vi "CPP_SpectraFit.vi"() -> (5 "Plug in titles":string[](array[string]), 7 "Plug in values":string[](array[string]))   [LabVIEW 2020]
uses:
  <vilib>/Analysis/2dsp.llb/Integral Method.ctl
  Controls/Instrument_Array.ctl
  Controls/Post_Process.ctl
  Controls/Graph_Type.ctl
  <vilib>/Analysis/8numeric.llb/1D Numeric Integration.vi
  Globals/Meas_global.vi
  <vilib>/Analysis/NI_AALPro.lvlib
  <vilib>/Analysis/NI_AALBase.lvlib
panel:
  out "Av Sampling Rate":dbl
  out "mean":dbl format="%0.2f"
  out "variance":dbl format="%.4f"
  out "Integral":dbl format="%0.4f"
  in  "integration method":T1 items=["Trapezoidal Rule", "Simpson's Rule", "Simpson's 3/8 Rule", "Bode Rule"]
  in  "Divider":i32(slide)=10 scale=1.0..100000.0 scale format="%#_6e"
  out "dF/ Hz":dbl
  in  "Show Smooth":bool=TRUE
  in  "Save Spectra?":bool
  in  "Desired number of samples per block":i32=32768
  out "Spectra":cluster{"Frequencies":dbl[], dbl[]}[](graph)
  in  "Averaging samples":i32=1 min=1 max=1000
  in  "Spectra Index (from ALL channels)":i32
  out "Waveform Graph":dbl[][](graph)
  in  "Channels to Plot":i32[](array[ring])=[0] items=["Pitot (URef)", "Mano (5HP1)", "Mano (5HP2)", "Mano (5HP3)", "Mano (5HP4)", "Mano (5HP5)", "HW (Uhf)", "Save Nothing"]
  # "Run this VI to update the channel names"
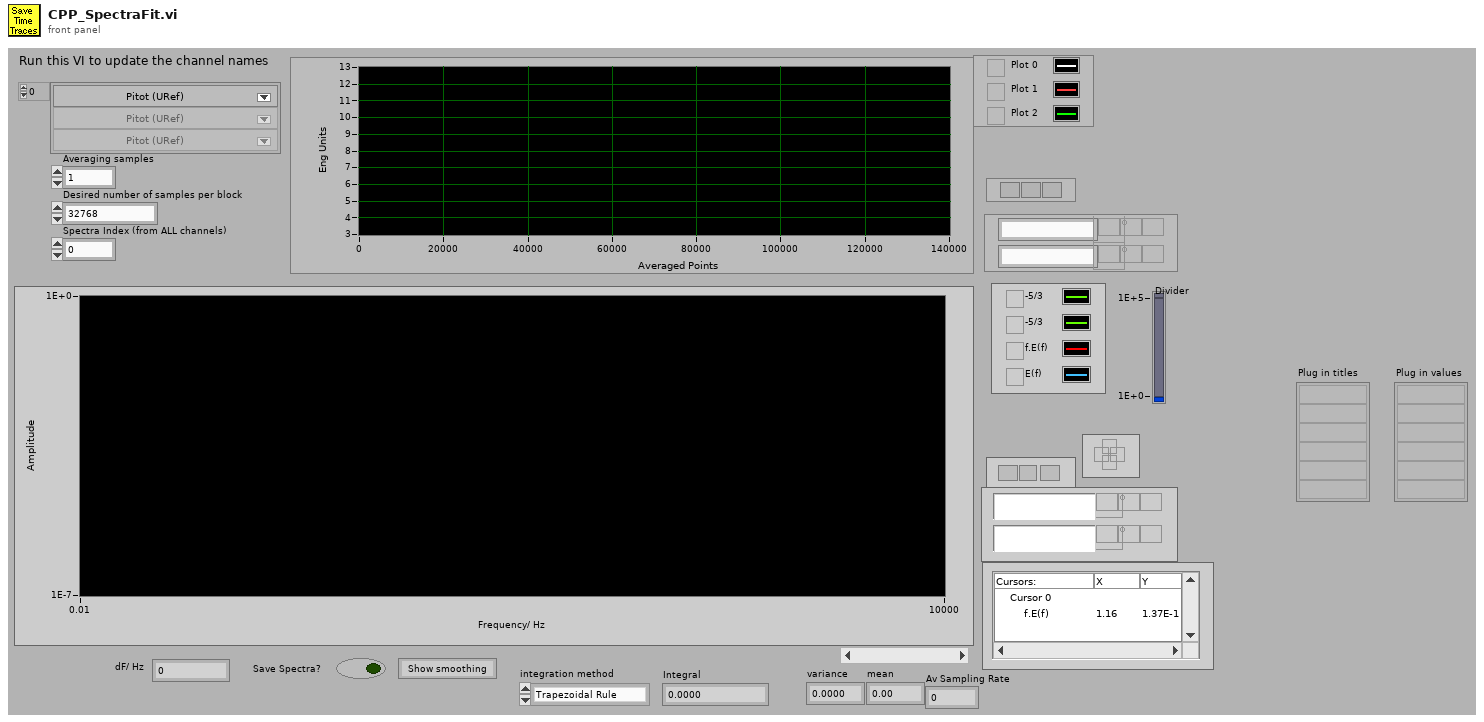
[diagram p1: front panel]
types:
  T1 = typedef "NI_AALPro.lvlib/Integral Method.ctl" = i32
  T2 = typedef "Analysis_info_cluster.ctl" = cluster{"Colour":u32, "Inst type":T3, "Inst name":string, "Symbol":string, "Code name":string, "Extra Info":string, "Inst Array":T4, "Extra Titles":string[], "Extra Values":string[], "U":dbl, "u^2":dbl, "u^3":dbl, "u^4":dbl, "Skew_u":dbl, "Kurt_u":dbl, "Sd Error in Mean":dbl, "% u'/U":dbl, "X":dbl, "Y":dbl, "Z":dbl, "Timescale integral Estimate":dbl, "Sd Error in Variance":dbl, "Calib File":path, "Calib Constants":dbl[], "Output Position":bool, "Stats":enum16{"None", "Basic", "Full"}, "Av Sampling Rate":dbl, "Av No of Samples":dbl, "Total Meas Time (s)":dbl, "ADAM Ch Name":string, "Max value":dbl, "Min value":dbl, "Req Sample Rate Hz":dbl, "Sync Delay Time (s)":dbl, "Ch No":i16, "Device":string, "Use Latest Calib":bool, "Port":string, "Metadata Ch Names":string[], "Metadata Ch Values":string[]}
  T3 = typedef "Inst_type.ctl" = enum16{"Propeller anemometer", "Raw voltage", "Pressure Transducer", "Pitot-static tube", "Preston tube", "Hot wire", "Cross wire 1", "Cross wire 2", "Generic Linear", "Generic Polynomial", "Generic BackPoly", "Fast FID", "Thermocouple", "Cold wire", "Pulsed Wire", "LDA Vel", "LDA Tran time", "LDA Arr time", "Microphone"}
  T4 = typedef "Instrument_Array.ctl" = enum16{"PWA", "LDA", "Analogue"}
  T5 = typedef "Post_Process.ctl" = enum16{"Take New Data", "Post Process Raw Data File"}
  T6 = typedef "Graph_Type.ctl" = enum16{"Show no graph", "Voltage trace", "Velocity trace", "Vel histogram", "Spectrum", "f.E(f) v Log f", "Auto-Corr"}
  T7 = cluster{"Plot 1":u16, "Plot 2":u16, "Save graph":u16, "Plot Type":T6}
  T8 = typedef "Time_Trace_Cluster.ctl" = cluster{"Weighting":dbl[], "Time (s)":dbl[], "Voltage":dbl[], "Eng Values":dbl[]}
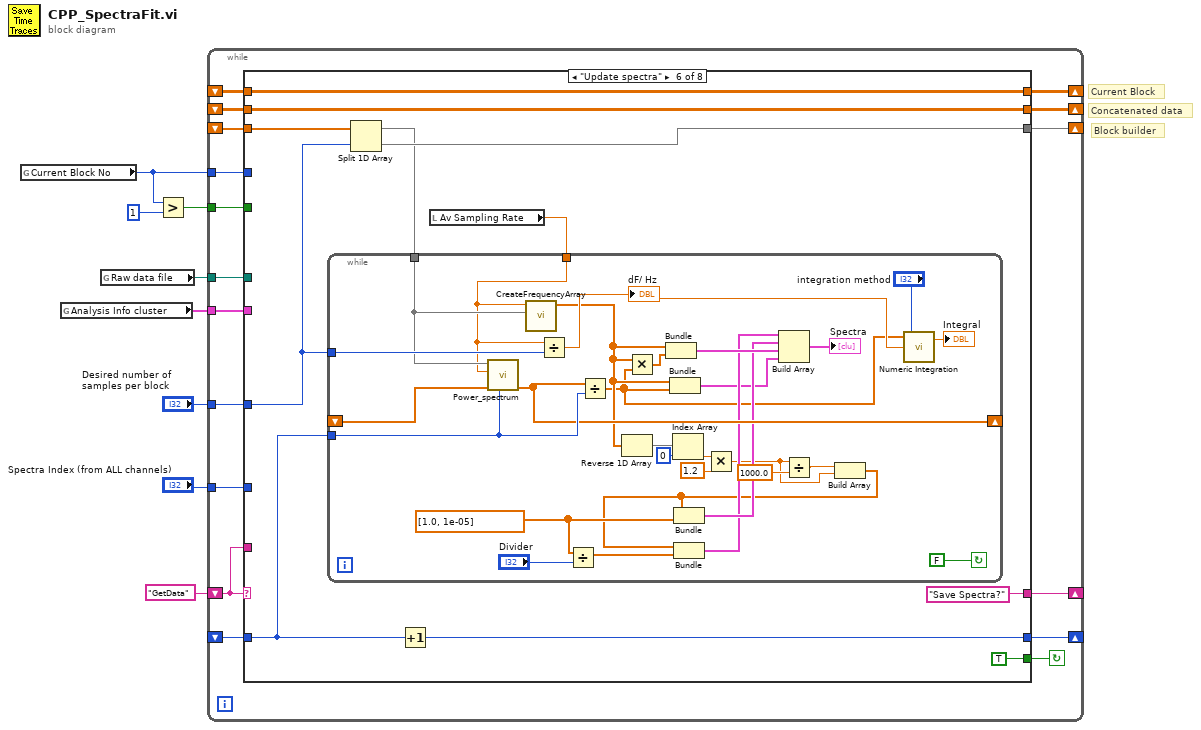
[diagram p0: block diagram]
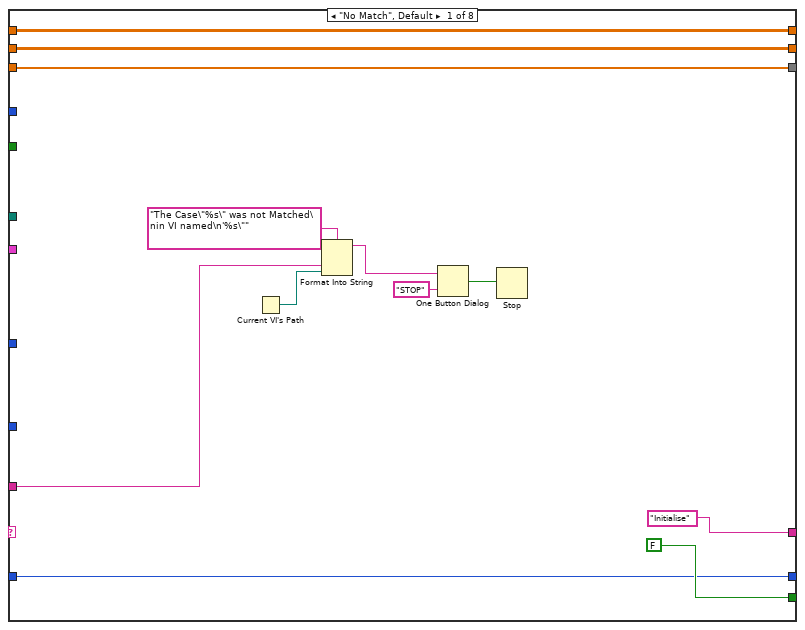
[diagram p2: hidden frame]
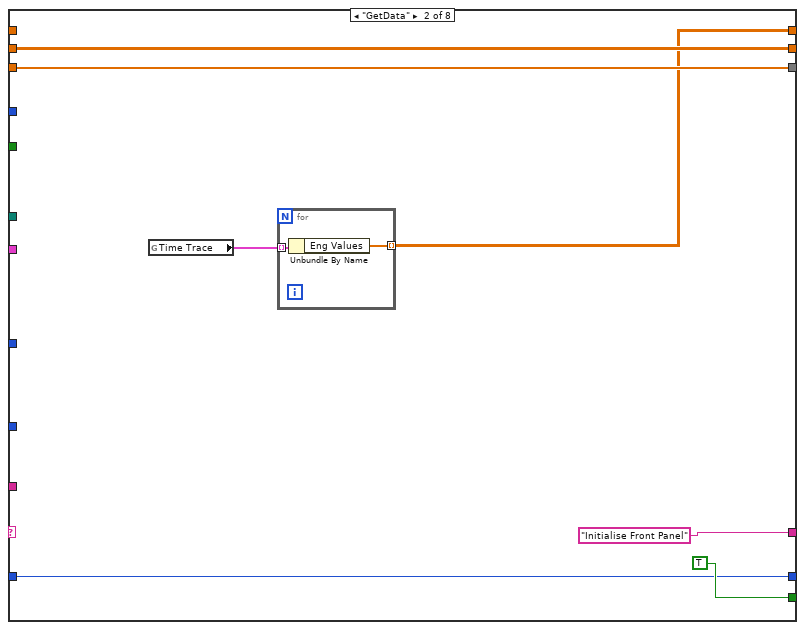
[diagram p3: hidden frame]
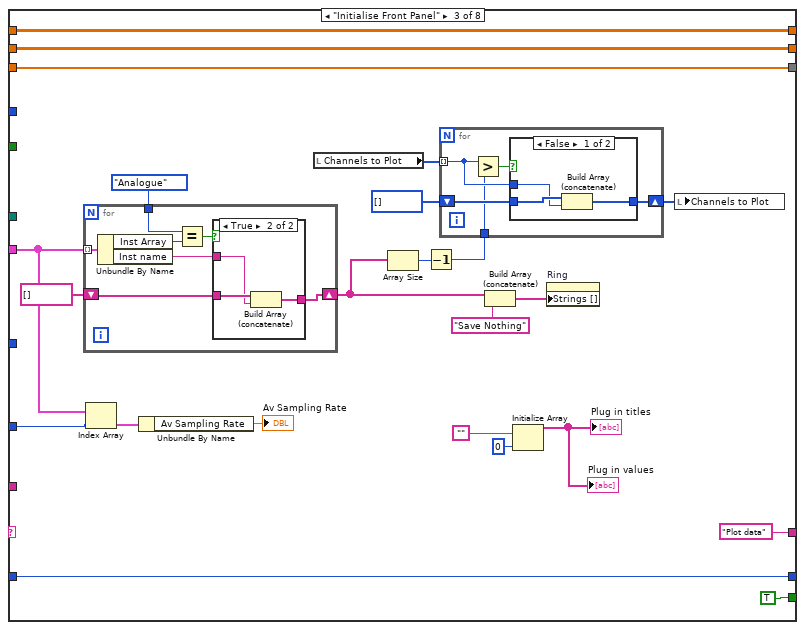
[diagram p4: hidden frame]
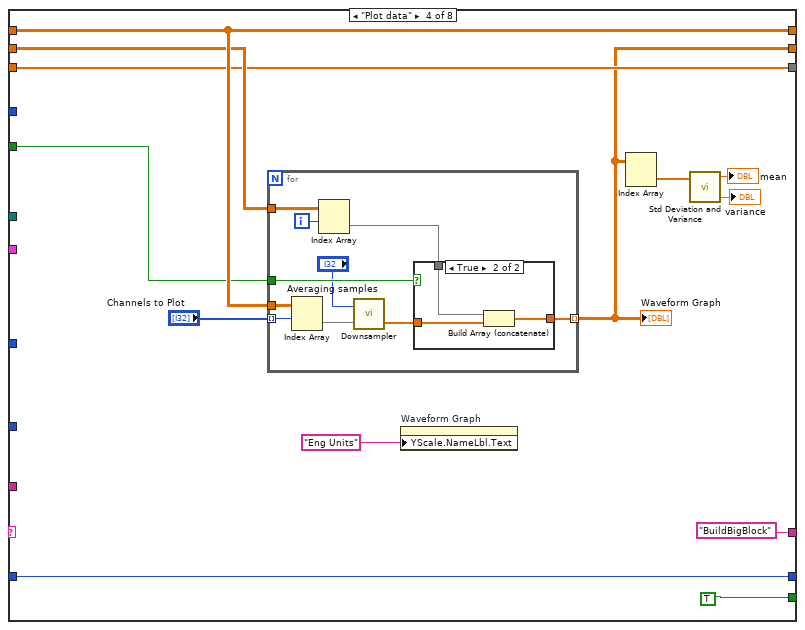
[diagram p7: hidden frame]
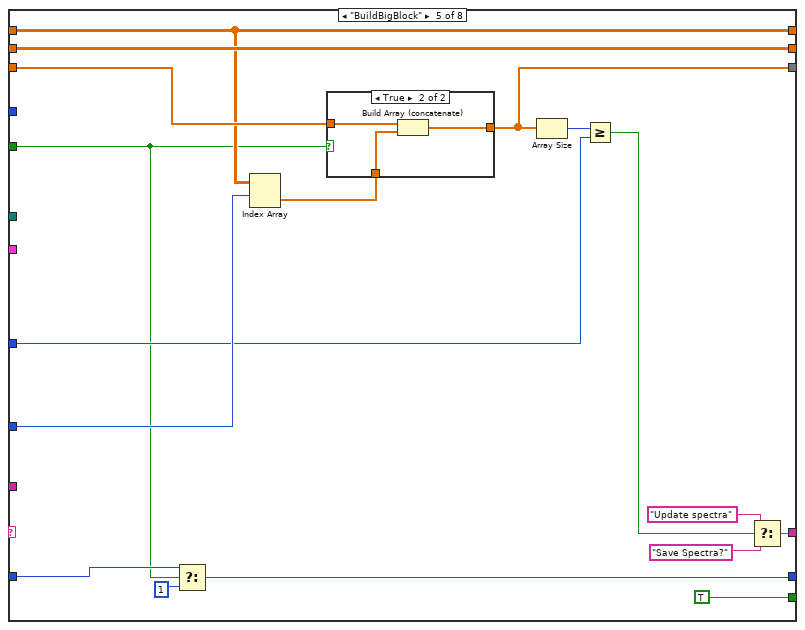
[diagram p9: hidden frame]
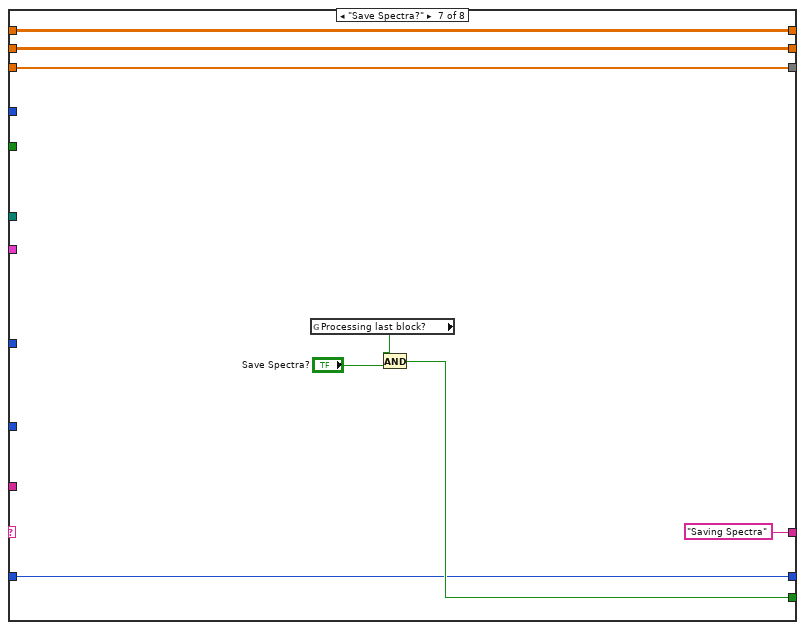
[diagram p11: hidden frame]
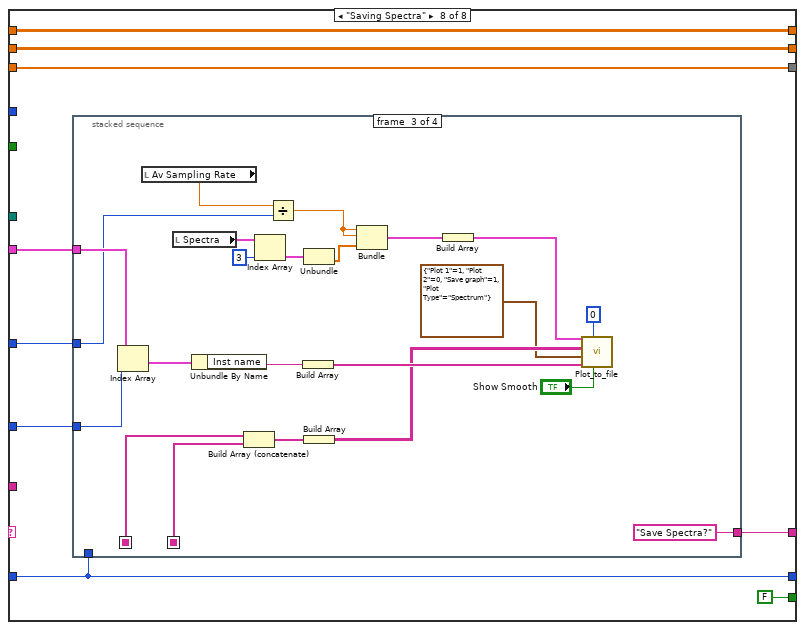
[diagram p12: hidden frame]
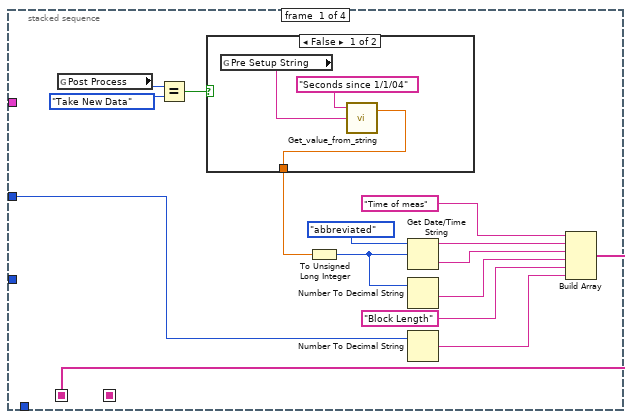
[diagram p13: hidden frame]
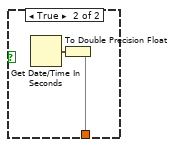
[diagram p14: hidden frame]
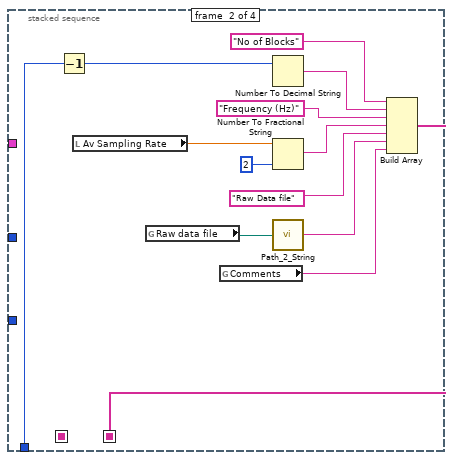
[diagram p15: hidden frame]
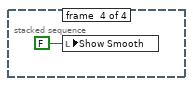
[diagram p16: hidden frame]
diagram:
  # "Block builder"
  # "Concatenated data"
  # "Current Block"
  n1 = global read "Meas_global.vi" "Current Block No"() -> (w5:i32)
  n2 = global read "Meas_global.vi" "Analysis Info cluster"() -> (w4:T2[])
  n3 = global read "Meas_global.vi" "Raw data file"() -> (w7:path)
  n4 = Greater?(x=w5, y=1) -> (0:w3:bool)
  n5 = while {
    shift-left: "GetData" -> [w23]
    shift-right: [w24] -> _
    tunnel: w7 -> [w22]
    tunnel: w3 -> [w21]
    tunnel: w5 -> [w20]
    tunnel: w4 -> [w19]
    shift-right: [w18] -> _
    shift-left: _ -> [w17]
    shift-right: [w15] -> _
    shift-left: _ -> [w16]
    shift-right: [w13] -> _
    shift-left: _ -> [w14]
    tunnel: "Desired number of samples per block" -> [w12]
    tunnel: "Spectra Index (from ALL channels)" -> [w11]
    shift-right: [w10] -> _
    shift-left: _ -> [w9]
    stop <- w25 continue-if-true
    n6 = case shown="\"Update spectra\"" w23 {
      tunnel: [FALSE TRUE TRUE TRUE ("Calculate Spectra and Histogram?") TRUE ("Calculate Spectra and Histogram?") TRUE ("Calculate Spectra and Histogram?") w179 FALSE ("Calculate Spectra and Histogram?")] -> w25
      tunnel: ["Initialise" "Initialise Front Panel" "Plot data" "BuildBigBlock" ("t") w118 "Save Spectra?" "Saving Spectra" w192] -> w24
      tunnel: w23 -> [w32 _ _ _ _ _ _ _]
      tunnel: w22 -> [_ _ _ _ _ _ _ _]
      tunnel: w21 -> [_ _ _ w100 w121 _ _ _]
      tunnel: w20 -> [_ _ _ _ _ _ _ _]
      tunnel: w19 -> [_ _ w50 _ _ _ _ w190]
      tunnel: [w29 w38 w59 w102 w131 w147 w184 w193] -> w18
      tunnel: w17 -> [w29 _ w59 w102 w131 w147 w184 w193]
      tunnel: w16 -> [w28 w42 w58 w101 w132 w148 w185 w194]
      tunnel: [w28 w42 w58 w93 w132 w148 w185 w194] -> w15
      tunnel: w14 -> [w27 w41 w55 w97 w133 w146 w182 w191]
      tunnel: [w27 w41 w55 w97 w129 w145 w182 w191] -> w13
      tunnel: w12 -> [_ _ _ _ w125 w141 _ w187]
      tunnel: w11 -> [_ _ w49 _ w127 _ _ w189]
      tunnel: [w26 w40 w54 w96 w122 w139 w178 w186] -> w10
      tunnel: w9 -> [w26 w40 w54 w96 w123 w140 w178 w186]
      frame "No Match", Default {
        n7 = Current VI's Path() -> (path=w31:path)
        n8 = Format Into String(format string="The Case\"%s\" was not Matched\nin VI named\n'%s\"" ("Format String"), w32, w31) -> (resulting string=w35:string)  [unwired: 2 in, 1 out]
        n9 = One Button Dialog(message=w35, button name ("OK")="STOP") -> (true=w33:bool)
        n10 = Stop(stop? (T)=w33) -> ()
      }
      frame "GetData" {
        n11 = global read "Meas_global.vi" "Time Trace"() -> (w39:T8[])
        n12 = for {
          tunnel: w39 -> [w46] mode=indexing
          tunnel: [w45] -> w38 mode=indexing
          n13 = Unbundle By Name(w46) -> ("Eng Values"=w45:dbl[])
        }
      }
      frame "Initialise Front Panel" {
        n14 = for {
          tunnel: Instrument_Array."Analogue" ("Inst Array") -> [w75]
          tunnel: w50 -> [w74] mode=indexing
          shift-right: [w71] -> w53
          shift-left: string[] [] -> [w72]
          n15 = Unbundle By Name(w74) -> ("Inst Array"=w76:T4, "Inst name"=w70:string)
          n16 = Equal?(x=w75, y=w76) -> (x = y?=w73:bool)
          n17 = case shown="True" w73 {
            tunnel: w72 -> [w77 w80]
            tunnel: [w77 w79] -> w71
            tunnel: w70 -> [_ w78]
            frame False {
            }
            frame True {
              n18 = Build Array (concatenate)(w80, w78) -> (w79:string[])
            }
          }
        }
        n19 = Index Array(array=w50, index=w49) -> (element=w48:T2)
        n20 = Unbundle By Name(w48) -> ("Av Sampling Rate"=→"Av Sampling Rate":dbl)
        n21 = local read "Channels to Plot"() -> (w66:i32[])
        n22 = Array Size(array=w53) -> (size(s)=w61:i32)
        n23 = Decrement(x=w61) -> (x-1=w60:i32)
        n24 = for {
          tunnel: w66 -> [w82] mode=indexing
          shift-right: [w83] -> w64
          shift-left: i32[] [] -> [w84]
          tunnel: w60 -> [w81]
          n25 = Greater?(x=w82, y=w81) -> (0:w85:bool)
          n26 = case shown="False" w85 {
            tunnel: w84 -> [w88 w89]
            tunnel: [w87 w89] -> w83
            tunnel: w82 -> [w86 _]
            frame False {
              n27 = Build Array (concatenate)(w88, w86) -> (w87:i32[])
            }
            frame True {
            }
          }
        }
        n28 = Build Array (concatenate)(w53, "Save Nothing") -> (w62:string[])
        n29 = Initialize Array("", 0) -> (→"Plug in values" →"Plug in titles":string[])
        n30 = property on="Ring" class="Ring (strict)"("Strings []"=w62) -> ()  [unwired: 2 in, 2 out]
        n31 = local write "Channels to Plot"(w64) -> ()
      }
      frame "Plot data" {
        n32 = for {
          tunnel: w102 -> [w112]
          tunnel: "Channels to Plot" -> [w111] mode=indexing
          tunnel: w101 -> [w108]
          tunnel: [w109] -> w93 mode=indexing
          tunnel: w100 -> [w110]
          i -> [w107]
          n33 = Index Array(array=w112, index (row)=w111) -> (element=w105:dbl[])  [unwired: 1 in]
          n34 = Index Array(array=w108, index (row)=w107) -> (element=w106:dbl[])  [unwired: 1 in]
          n35 = call "Downsampler.vi"("Input Array"=w105, "Averaging samples"="Averaging samples") -> ("Downsampled Array"=w104:dbl[])  [unwired: 1 out]
          n36 = case shown="True" w110 {
            tunnel: w106 -> [_ w116]
            tunnel: w104 -> [w113 w115]
            tunnel: [w113 w114] -> w109
            frame False {
            }
            frame True {
              n37 = Build Array (concatenate)(w116, w115) -> (w114:dbl[])
            }
          }
        }
        "Waveform Graph" <- w93
        n38 = property on="Waveform Graph" class="WFGraph (strict)"("YScale.NameLbl.Text"="Eng Units") -> ()  [unwired: 2 in, 2 out]
        n39 = Index Array(array=w93) -> (element=w92:dbl[])  [unwired: 2 in]
        n40 = call <vilib>:"Std Deviation and Variance.vi"("X"=w92) -> ("mean"=→"mean":dbl, "variance"=→"variance":dbl)  [unwired: 1 in, 1 out]
      }
      frame "BuildBigBlock" {
        n41 = Select(t=w123, s=w121, f=1) -> (s? t:f=w122:i32)
        n42 = Index Array(array=w131, index (row)=w127) -> (element=w130:dbl[])  [unwired: 1 in]
        n43 = case shown="True" w121 {
          tunnel: w133 -> [_ w137]
          tunnel: [w134 w136] -> w129
          tunnel: w130 -> [w134 w135]
          frame False {
          }
          frame True {
            n44 = Build Array (concatenate)(w137, w135) -> (w136:dbl[])
          }
        }
        n45 = Array Size(array=w129) -> (size(s)=w128:i32)
        n46 = Greater Or Equal?(x=w128, y=w125) -> (x >= y?=w117:bool)
        n47 = Select(t="Update spectra", s=w117, f="Save Spectra?") -> (s? t:f=w118:string)
      }
      frame "Update spectra" {
        n48 = Split 1D Array(array=w146, index=w141) -> (first subarray=w142:dbl[], second subarray=w145:dbl[])
        n49 = Increment(x=w140) -> (x+1=w139:i32)
        n50 = local read "Av Sampling Rate"() -> (w138:dbl)
        n51 = while {
          shift-left: _ -> [w173]
          shift-right: [w174] -> _
          tunnel: w142 -> [w172]
          tunnel: w140 -> [w176]
          tunnel: w141 -> [w175]
          tunnel: w138 -> [w149]
          stop <- FALSE continue-if-true
          w167 = dbl[] [1.0, 1e-05]
          n52 = call "Power_spectrum.vi"("Block No"=w176, "Spectrum input array"=w173, "Sampling frequency"=w149, "U"=w172) -> ("Spectrum Accumulator array"=w174:dbl[])  [unwired: 1 in, 3 out]
          n53 = call "CreateFrequencyArray.vi"("Signal"=w172, "Actual Sampling rate (Hz)"=w149) -> ("Frequencies"=w153:dbl[])  [unwired: 9 in]
          n54 = Divide(x=w149, y=w175) -> (x/y=w154:dbl)
          "dF/ Hz" <- w154
          n55 = Divide(x=w167, y="Divider") -> (x/y=w168:dbl[])
          n56 = Divide(x=w174, y=w176) -> (x/y=w150:dbl[])
          n57 = Reverse 1D Array(array=w153) -> (reversed array=w162:dbl[])
          n58 = Multiply(x=w153, y=w150) -> (x*y=w164:dbl[])
          n59 = Bundle("Frequencies"=w153, w164) -> (w170:cluster{"Frequencies":dbl[], dbl[]})  [unwired: 1 in]
          n60 = Bundle("Frequencies"=w153, w150) -> (w163:cluster{"Frequencies":dbl[], dbl[]})  [unwired: 1 in]
          n61 = Index Array(array=w162, index=0) -> (element=w160:dbl)
          n62 = Multiply(x=w160, y=1.2) -> (x*y=w156:dbl)
          n63 = Divide(x=w156, y=1000.0) -> (x/y=w157:dbl)
          n64 = Build Array(w157, w156) -> (w155:dbl[])
          n65 = Bundle(w155, w167) -> (w169:cluster{dbl[], dbl[]})  [unwired: 1 in]
          n66 = Bundle(w155, w168) -> (w165:cluster{dbl[], dbl[]})  [unwired: 1 in]
          n67 = Build Array(w165, w169, w170, w163) -> (→"Spectra":cluster{"Frequencies":dbl[], dbl[]}[])
          n68 = call-poly <vilib>:"Numeric Integration.vi"("integration method"="integration method", "dt"=w154, "Input Array"=w150) -> ("result"=→"Integral":dbl)  [unwired: 1 out]
        }
      }
      frame "Save Spectra?" {
        n69 = global read "Meas_global.vi" "Processing last block?"() -> (w180:bool)
        n70 = And(x=w180, y="Save Spectra?") -> (x .and. y?=w179:bool)
      }
      frame "Saving Spectra" {
        n71 = stacked-sequence {
          seq-local: [w198 _ _ _] -> [_ _ w240 _]
          seq-local: [_ w219 _ _] -> [_ _ w239 _]
          tunnel: [_ _ "Save Spectra?" _] -> w192
          tunnel: w190 -> [_ _ w246 _]
          tunnel: w189 -> [_ _ w245 _]
          tunnel: w187 -> [w196 _ w232 _]
          tunnel: w186 -> [_ w217 _ _]
          frame #0 {
            n72 = global read "Meas_global.vi" "Post Process"() -> (w200:T5)
            n73 = Equal?(x=w200, y=Post_Process."Take New Data" ("Post Process")) -> (x = y?=w201:bool)
            n74 = case shown="False" w201 {
              tunnel: [w209 w213] -> w202
              frame False {
                n75 = global read "Meas_global.vi" "Pre Setup String"() -> (w210:string)
                n76 = call "Get_value_from_string.vi"("Input string"=w210, "Variable name"="Seconds since 1/1/04") -> ("Value"=w209:dbl)  [unwired: 1 in, 1 out]
              }
              frame True {
                n77 = Get Date/Time In Seconds() -> (seconds since 1Jan1904=w212:timestamp)
                n78 = To Double Precision Float(number=w212) -> (double precision float=w213:dbl)
              }
            }
            n79 = To Unsigned Long Integer(number=w202) -> (unsigned 32bit integer=w206:u32)
            n80 = Get Date/Time String(date format (0)=enum16{"short", "long", "abbreviated"}."abbreviated", seconds (now)=w206) -> (date string=w204:string, time string=w205:string)  [unwired: 1 out]
            n81 = Number To Decimal String(number=w206) -> (decimal integer string=w207:string)  [unwired: 1 out]
            n82 = Number To Decimal String(number=w196) -> (decimal integer string=w195:string)  [unwired: 1 out]
            n83 = Build Array("Time of meas", w204, w205, w207, "Block Length" ("element"), w195) -> (w198:string[])
          }
          frame #1 {
            n84 = Decrement(x=w217) -> (x-1=w216:i32)
            n85 = local read "Av Sampling Rate"() -> (w214:dbl)
            n86 = global read "Meas_global.vi" "Raw data file"() -> (w225:path)
            n87 = global read "Meas_global.vi" "Comments"() -> (w224:string)
            n88 = Number To Decimal String(number=w216) -> (decimal integer string=w215:string)  [unwired: 1 out]
            n89 = Number To Fractional String(number=w214, precision (6)=i16 2) -> (F-format string=w222:string)  [unwired: 2 out]
            n90 = call "Path_2_String.vi"("Real Path"=w225) -> ("Path String"=w226:string)
            n91 = Build Array("No of Blocks", w215, "Frequency (Hz)", w222, "Raw Data file", w226, w224) -> (w219:string[])
          }
          frame #2 {
            n92 = Index Array(array=w246, index=w245) -> (element=w244:T2)
            n93 = local read "Av Sampling Rate"() -> (w227:dbl)
            n94 = local read "Spectra"() -> (w235:cluster{"Frequencies":dbl[], dbl[]}[])
            n95 = Unbundle By Name(w244) -> ("Inst name"=w243:string)
            n96 = Build Array (concatenate)(w240, w239) -> (w238:string[])
            n97 = Index Array(array=w235, index=3) -> (element=w233:cluster{"Frequencies":dbl[], dbl[]})
            n98 = Divide(x=w227, y=w232) -> (x/y=w230:dbl)
            n99 = Build Array(w243) -> (w242:string[])
            n100 = Unbundle(w233) -> (w231:dbl[])  [unwired: 1 out]
            n101 = Build Array(w238) -> (w237:string[][])
            n102 = Bundle(w230, w230, w231) -> (w229:cluster{dbl, dbl, dbl[]})  [unwired: 1 in]
            n103 = Build Array(w229) -> (w228:cluster{dbl, dbl, dbl[]}[])
            n104 = call "Plot_to_file.vi"("Show Smooth"="Show Smooth", "Start trace No"=0, "Trace names"=w242, "Graph"=T7 {"Plot 1"=1, "Plot 2"=0, "Save graph"=1, "Plot Type"=enum."Spectrum"}, "Plot file label"=w237, "Plot data"=w228) -> ()  [unwired: 6 out]
          }
          frame #3 {
            n105 = local write "Show Smooth"(FALSE ("Show Smooth")) -> ()
          }
        }
      }
    }
  }
